vi "Read Pins.vi"(8 "error in (no error)":errorcluster, 11 "Stage Actor.lvlib:Stage.lvclass":refnum<class "Stage.lvclass">) -> (0 "error out":errorcluster, 3 "Stage Actor.lvlib:Stage.lvclass":refnum<class "Stage.lvclass">)   [LabVIEW 2018, in "Stage Actor.lvlib" / "Stage.lvclass"]
uses:
  Stage.lvclass
  C:/Program Files/National Instruments/LabVIEW 2018/vi.lib/ActorFramework/Actor/Actor.lvclass
  Stage.lvclass/Stage.ctl
  <vilib>/ActorFramework/Actor/Actor.lvclass/Actor.ctl
  ADM/Main Messages/Set Flow Msg/Set Flow Msg.lvclass/Set Flow Msg.ctl
  <vilib>/ActorFramework/Message Enqueuer/Message Enqueuer.lvclass/Message Enqueuer.ctl
  <vilib>/ActorFramework/Message Enqueuer/Enqueue.vi
  ADM/Main Messages/Set Flow Msg/Set Flow Msg.lvclass
  C:/Program Files/National Instruments/LabVIEW 2018/vi.lib/ActorFramework/Message/Message.lvclass
  <vilib>/ActorFramework/Message Priority Queue/Priority Enqueue.vi
  <instrlib>/Zaber A Series/Zaber A Series.lvlib
  <vilib>/ActorFramework/Actor/Actor.lvclass
  ADM/Main Messages/Switch Tool Msg/Switch Tool Msg.lvclass
panel:
  out "Digital Input Pins":bool[](array[boolean])
  out "Analog Inputs":dbl[](array[numeric])
  out "Digital Output Pins":bool[](array[boolean])
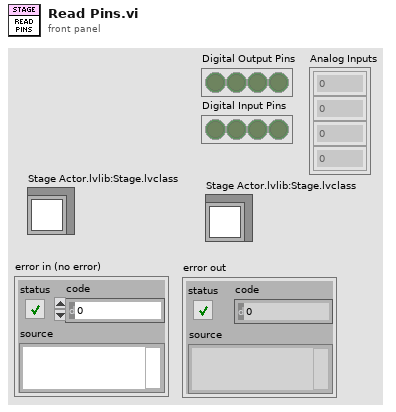
[diagram p1: front panel]
types:
  T1 = cluster{"Digital Output Pins[0]":bool, "Digital Output Pins[1]":bool, "Digital Output Pins[2]":bool, "Digital Output Pins[3]":bool, "Digital Output Pins[4]":bool, "Digital Output Pins[5]":bool, "Digital Output Pins[6]":bool, "Digital Output Pins[7]":bool, "Digital Output Pins[8]":bool}
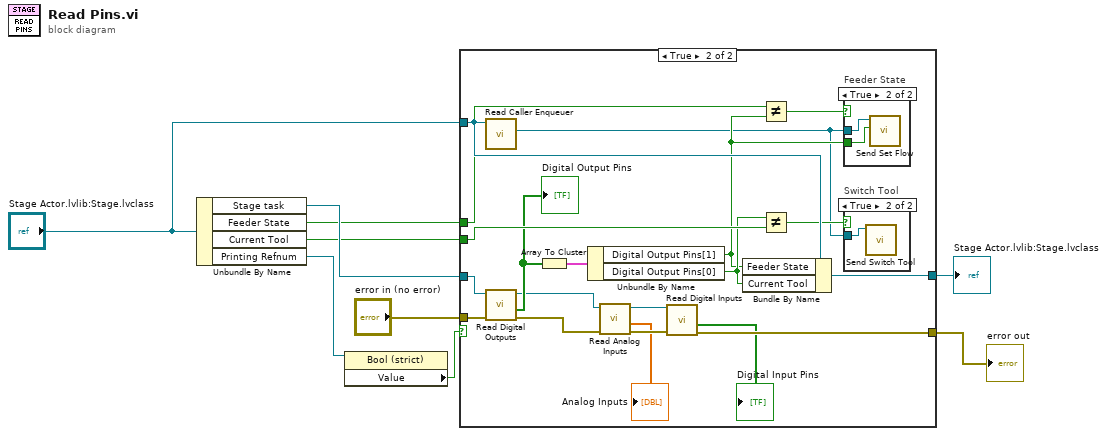
[diagram p0: block diagram]
diagram:
  n1 = Unbundle By Name("Stage Actor.lvlib:Stage.lvclass") -> ("Stage task"=w9:refnum<visa-resource-name>, "Feeder State"=w5:bool, "Current Tool"=w4:bool, "Printing Refnum"=w3:refnum<vi>)
  n2 = property class="Bool (strict)"(reference=w3) -> ("Value"=w2:bool)  [unwired: 1 in, 2 out]
  n3 = case shown="True" w2 {
    tunnel: w9 -> [_ w31]
    tunnel: "error in (no error)" -> [w10 w30]
    tunnel: "Stage Actor.lvlib:Stage.lvclass" -> [w11 w29]
    tunnel: [w11 w28] -> w6
    tunnel: w5 -> [_ w27]
    tunnel: w4 -> [_ w26]
    tunnel: [w10 w17] -> w1
    frame False {
    }
    frame True {
      n4 = call <vilib>:"Read Caller Enqueuer.vi"("Actor"=w29) -> ("Caller Enqueuer"=w12:refnum<class "Message Enqueuer.lvclass">)  [unwired: 10 in]
      n5 = call <instrlib>:"Read Digital Outputs.vi"("error in (no error)"=w30, "VISA resource name"=w31) -> ("error out"=w19:errorcluster, "Digital Output Pins"=w24:bool[], "VISA resource name out"=w16:refnum<visa-resource-name>)  [unwired: 7 in]
      "Digital Output Pins" <- w24
      n6 = Array To Cluster(array=w24) -> (cluster=w25:T1)
      n7 = Unbundle By Name(w25) -> ("Digital Output Pins[1]"=w20:bool, "Digital Output Pins[0]"=w21:bool)
      n8 = call <instrlib>:"Read Analog Inputs.vi"("error in (no error)"=w19, "VISA resource name"=w16) -> ("error out"=w18:errorcluster, "Analog Inputs"=→"Analog Inputs":dbl[], "VISA resource name out"=w15:refnum<visa-resource-name>)  [unwired: 7 in]
      n9 = call <instrlib>:"Read Digital Inputs.vi"("error in (no error)"=w18, "VISA resource name"=w15) -> ("error out"=w17:errorcluster, "Digital Input Pins"=→"Digital Input Pins":bool[])  [unwired: 7 in, 1 out]
      n10 = Bundle By Name(cluster=w29, "Feeder State"=w20, "Current Tool"=w21) -> (w28:refnum<class "Stage.lvclass">)
      n11 = Not Equal?(x=w27, y=w20) -> (x != y?=w22:bool)
      n12 = Not Equal?(x=w21, y=w26) -> (x != y?=w23:bool)
      n13 = case "Feeder State" shown="True" w22 {
        tunnel: w12 -> [_ w34]
        tunnel: w20 -> [_ w33]
        frame False {
        }
        frame True {
          n14 = call "Send Set Flow.vi"("State"=w33, "Message Enqueuer in"=w34) -> ()  [unwired: 8 in, 2 out]
        }
      }
      n15 = case "Switch Tool" shown="True" w23 {
        tunnel: w12 -> [_ w32]
        frame False {
        }
        frame True {
          n16 = call "Send Switch Tool.vi"("Message Enqueuer in"=w32) -> ()  [unwired: 9 in, 2 out]
        }
      }
    }
  }
  "Stage Actor.lvlib:Stage.lvclass" <- w6
  "error out" <- w1
